vi "Gen Filter Statement.vi"(8 "error in":errorcluster, 10 "Columns":string[](array[string]), 11 "Filter Cluster in":refnum<vi>) -> (0 "error out":errorcluster, 3 "Filter String":string)   [LabVIEW 2021, in "EDT SQLite+.lvlib"]
uses:
  EDT SQLite+.lvlib
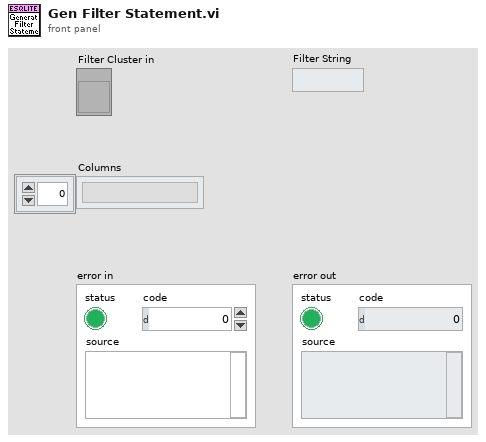
[diagram p1: front panel]
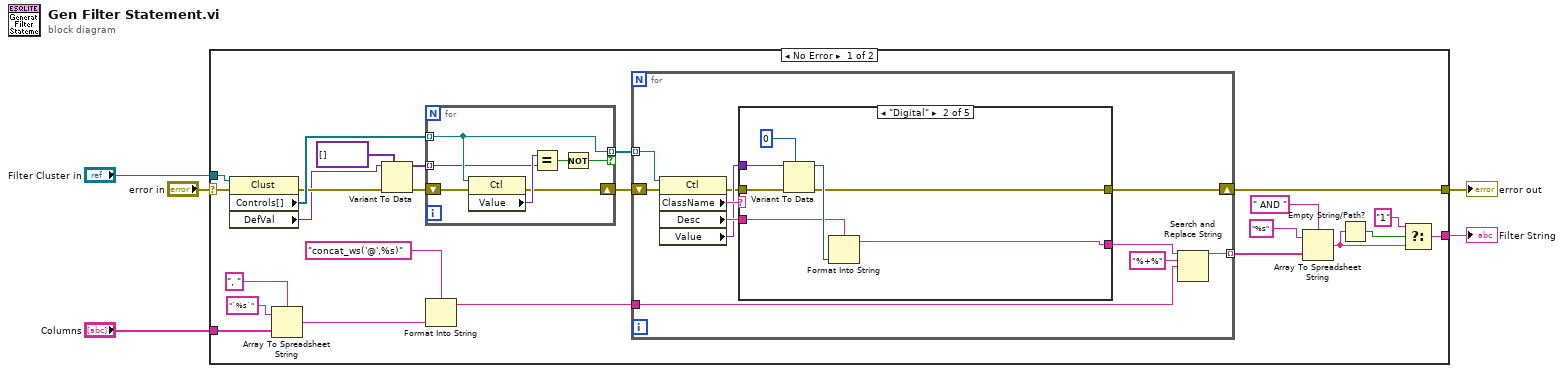
[diagram p0: block diagram]
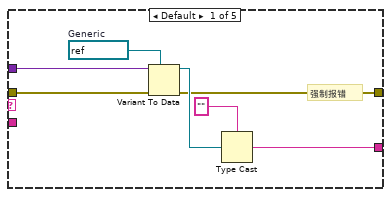
[diagram p2: hidden frame]
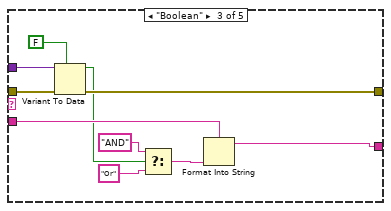
[diagram p3: hidden frame]
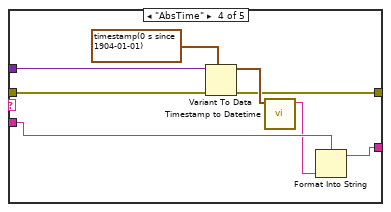
[diagram p4: hidden frame]
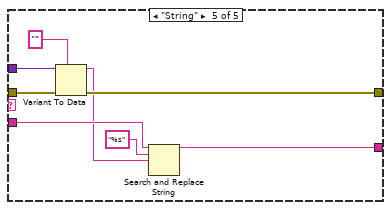
[diagram p5: hidden frame]
diagram:
  n1 = case shown="No Error" "error in" {
    selector: "error in" -> [w24 w88]
    tunnel: "Filter Cluster in" -> [w27 _]
    tunnel: [w20 w88] -> w4
    tunnel: [w6 _] -> w1
    tunnel: "Columns" -> [w16 _]
    frame No Error {
      n2 = property on="Property Node" class="Clust"(reference=w27, error in=w24) -> (error out=w23:errorcluster, "Controls[]"=w25:refnum<vi>[], "DefVal"=w10:variant)  [unwired: 1 out]
      n3 = Array To Spreadsheet String(delimiter (Tab)=", ", array=w16, 3:"`%s`" ("format string")) -> (spreadsheet string=w13:string)
      n4 = Variant To Data(error in=w23, type=variant[] [], Variant=w10) -> (data=w29:variant[], error out=w22:errorcluster)
      n5 = for {
        tunnel: w25 -> [w86] mode=indexing
        tunnel: [w86] -> w26 mode=indexing if=w87
        tunnel: w29 -> [w84] mode=indexing
        shift-right: [w81] -> w21
        shift-left: w22 -> [w82]
        n6 = property class="Ctl"(reference=w86, error in=w82) -> (error out=w81:errorcluster, "Value"=w85:variant)  [unwired: 1 out]
        n7 = Equal?(x=w85, y=w84) -> (x = y?=w83:bool)
        n8 = Not(x=w83) -> (.not. x?=w87:bool)
      }
      n9 = Format Into String(format string="concat_ws('@',%s)", w13) -> (resulting string=w11:string)  [unwired: 2 in, 1 out]
      n10 = for {
        tunnel: w26 -> [w40] mode=indexing
        tunnel: [w30] -> w17 mode=indexing
        shift-right: [w34] -> w20
        shift-left: w21 -> [w36]
        tunnel: w11 -> [w33]
        n11 = property class="Ctl"(reference=w40, error in=w36) -> (error out=w35:errorcluster, "ClassName"=w39:string, "Desc"=w38:string, "Value"=w37:variant)  [unwired: 1 out]
        n12 = case shown="\"Digital\"" w39 {
          tunnel: w38 -> [_ w51 w63 w70 w75]
          tunnel: w37 -> [w47 w54 w64 w72 w80]
          tunnel: w35 -> [w42 w50 w62 w69 w79]
          tunnel: [w43 w49 w61 w68 w78] -> w34
          tunnel: [w41 w48 w60 w65 w77] -> w32
          frame Default {
            w46 = refnum<vi> refnum  # Generic
            # "强制报错"
            n13 = Variant To Data(error in=w42, type=w46, Variant=w47) -> (data=w45:refnum<vi>, error out=w43:errorcluster)
            n14 = Type Cast(type="", x=w45) -> (*(type *) &x=w41:string)
          }
          frame "Digital" {
            n15 = Variant To Data(error in=w50, type=0, Variant=w54) -> (data=w52:i32, error out=w49:errorcluster)
            n16 = Format Into String(format string=w51, w52) -> (resulting string=w48:string)  [unwired: 2 in, 1 out]
          }
          frame "Boolean" {
            n17 = Variant To Data(error in=w62, type=FALSE, Variant=w64) -> (data=w58:bool, error out=w61:errorcluster)
            n18 = Select(t="AND" ("Desc"), s=w58, f="Or") -> (s? t:f=w55:string)
            n19 = Format Into String(format string=w63, w55) -> (resulting string=w60:string)  [unwired: 2 in, 1 out]
          }
          frame "AbsTime" {
            n20 = Variant To Data(error in=w69, type=timestamp(0 s since 1904-01-01), Variant=w72) -> (data=w71:timestamp, error out=w68:errorcluster)
            n21 = call "Timestamp to Datetime.vi"("Time Stamp"=w71) -> ("date/time string"=w66:string)  [unwired: 10 in]
            n22 = Format Into String(format string=w70, w66) -> (resulting string=w65:string)  [unwired: 2 in, 1 out]
          }
          frame "String" {
            n23 = Variant To Data(error in=w79, type="" ("format string"), Variant=w80) -> (data=w73:string, error out=w78:errorcluster)
            n24 = Search and Replace String(input string=w75, search string="%s", replace string=w73) -> (result string=w77:string)  [unwired: 5 in, 3 out]
          }
        }
        n25 = Search and Replace String(input string=w32, search string="%+%", replace string=w33) -> (result string=w30:string)  [unwired: 5 in, 3 out]
      }
      n26 = Array To Spreadsheet String(delimiter (Tab)=" AND ", array=w17, 3:"%s" ("format string")) -> (spreadsheet string=w8:string)
      n27 = Empty String/Path?(string/path=w8) -> (empty?=w9:bool)
      n28 = Select(t="1", s=w9, f=w8) -> (s? t:f=w6:string)
    }
    frame Error {
    }
  }
  "error out" <- w4
  "Filter String" <- w1
